vi "testAll.vi"(8 "error in (no error)":errorcluster) -> (0 "error out":errorcluster)   [LabVIEW 2018]
doc: "Run all the unit tests."
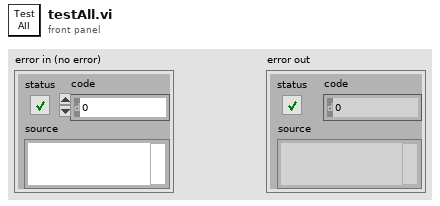
[diagram p1: front panel]
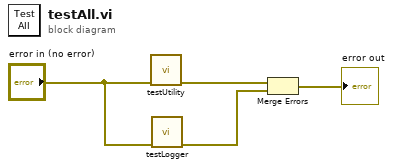
[diagram p0: block diagram]
diagram:
  n1 = call "testUtility.vi"("error in (no error)"="error in (no error)") -> ("error out"=w3:errorcluster)  [unwired: 10 in]
  n2 = call "testLogger.vi"("error in (no error)"="error in (no error)") -> ("error out"=w2:errorcluster)  [unwired: 10 in]
  n3 = Merge Errors(w3, w2) -> (→"error out":errorcluster)
